vi "starting_elements.get_quantity.vi"(11 "Snake in":refnum<class "Snake.lvclass">) -> (2 "Starting Elements":i32)   [LabVIEW 2020, in "Snake.lvclass"]
uses:
  Snake.lvclass
  Snake.lvclass/Snake.ctl
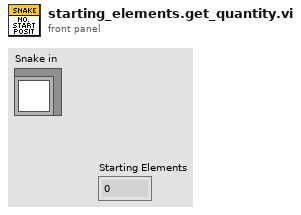
[diagram p1: front panel]
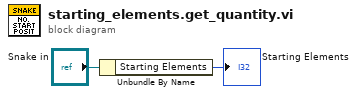
[diagram p0: block diagram]
diagram:
  n1 = Unbundle By Name("Snake in") -> ("Starting Elements"=→"Starting Elements":i32)
